vi "Update TDMS Tagged Packet Offsets.vi"(0 "llp tagged packet file path":path, 11 "error in":errorcluster) -> (4 "llp tagged packet file path out":path, 15 "error out":errorcluster)   [LabVIEW 2023, in "GettingStarted_Common_148X_Host.lvlib"]
uses:
  GettingStarted_Common_148X_Host.lvlib
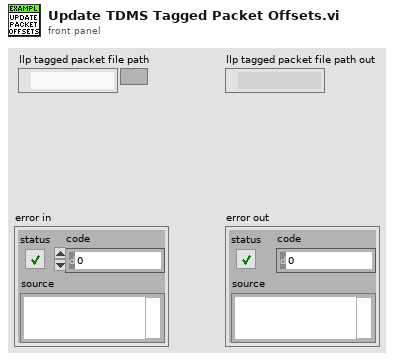
[diagram p1: front panel]
types:
  T1 = enum16{"open", "open or create", "create or replace", "create", "open (read-only)"}
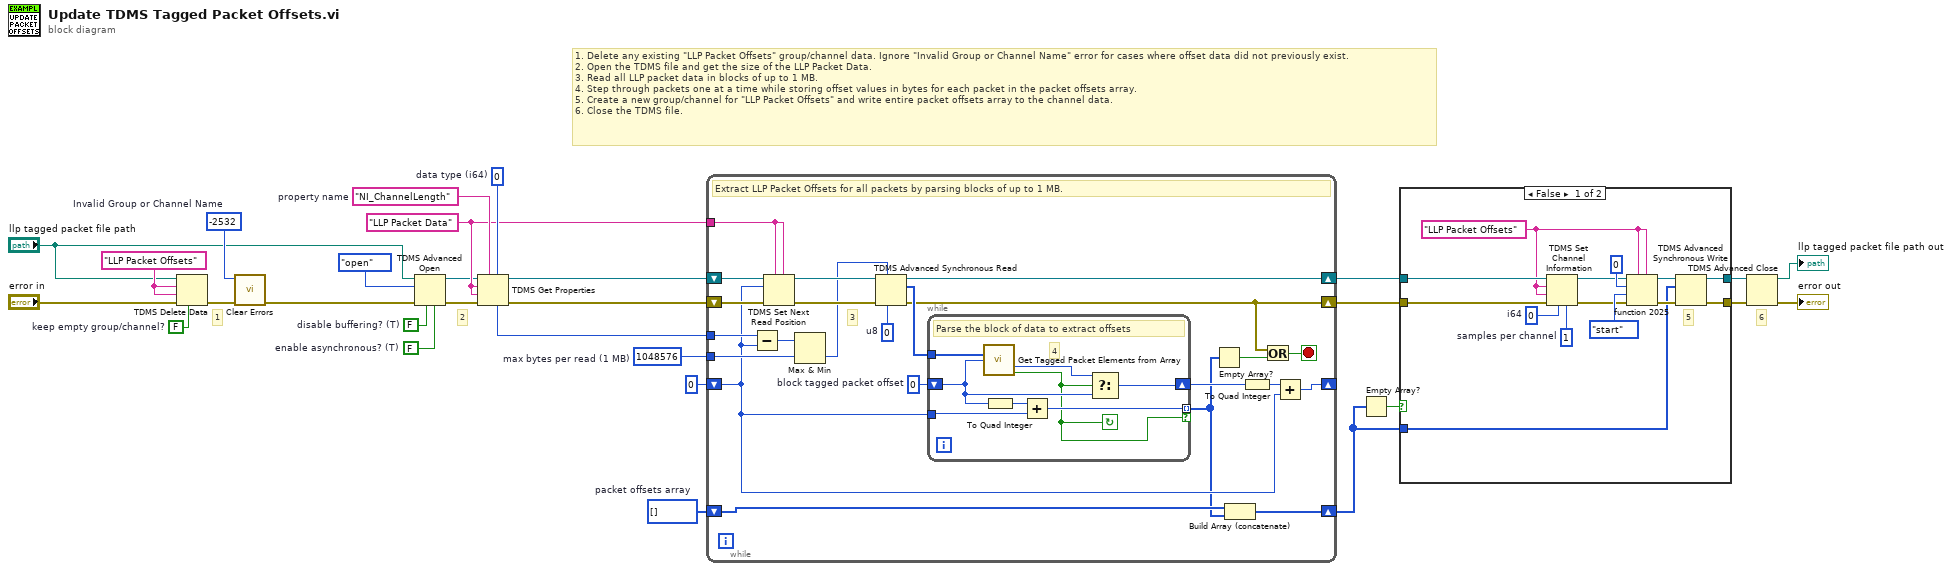
[diagram p0: block diagram]
diagram:
  w2 = -2532  # Invalid Group or Channel Name
  w5 = FALSE  # keep empty group/channel?
  w6 = "LLP Packet Offsets" ("channel and group name")
  w11 = i64[] []  # packet offsets array
  w23 = FALSE  # disable buffering? (T)
  w24 = FALSE  # enable asynchronous? (T)
  w25 = i64 1048576  # max bytes per read (1 MB)
  w28 = i64 0  # data type (i64)
  w29 = "NI_ChannelLength"  # property name
  w27 = "LLP Packet Data" ("channel and group name")
  # "6"
  # "2"
  # "1"
  # "1. Delete any existing \"LLP Packet Offsets\" group/channel data. Ignore \"Invalid Group or Channel Name\" error for cases where offset data did not previously exist.\n2. Open the TDMS file and get the size of the LLP Packet Data.\n3. Read all LLP packet data in blocks of up to 1 MB.\n4. Step through packets one at a time while storing offset values in bytes for each packet in the packet offsets array.\n5. Create a new group/channel for \"LLP Packet Offsets\" and write entire packet offsets array to the channel data.\n6. Close the TDMS file."
  n1 = TDMS Delete Data(6:w5, 8:"error in", 9:w6, 10:w6, 11:"llp tagged packet file path") -> (0:w4:errorcluster)  [unwired: 2 in, 1 out]
  n2 = call <vilib>:"Clear Errors.vi"("error in (no error)"=w4, "specific error code to clear (0: all)"=w2) -> ("error out"=w3:errorcluster)  [unwired: 4 in, 1 out]
  n3 = TDMS Advanced Open(4:w24, 6:w23, 8:w3, 10:T1."open" ("operation (0:open)"), 11:"llp tagged packet file path") -> (0:w13:errorcluster, 3:w12:refnum<k34>)  [unwired: 1 out]
  n4 = TDMS Get Properties(5:w28, 7:w29, 8:w13, 9:w27, 10:w27, 11:w12) -> (0:w19:errorcluster, 3:w18:refnum<k34>, 4:w26:i64)  [unwired: 3 out]
  n5 = while {
    shift-right: [w37] -> w16
    shift-left: w11 -> [w40]
    shift-right: [w36] -> _
    shift-left: i64 0 -> [w34]
    tunnel: w27 -> [w50]
    shift-right: [w31] -> w8
    shift-left: w19 -> [w51]
    shift-right: [w30] -> w9
    shift-left: w18 -> [w52]
    tunnel: w26 -> [w49]
    tunnel: w25 -> [w47]
    stop <- w38 stop-if-true
    w41 = u32 0  # block tagged packet offset
    w43 = u8 0  # u8
    # "3"
    # "Extract LLP Packet Offsets for all packets by parsing blocks of up to 1 MB."
    n6 = Subtract(x=w49, y=w34) -> (x-y=w48:i64)
    n7 = TDMS Set Next Read Position(5:w50, 7:w50, 8:w51, 10:w34, 11:w52) -> (0:w45:errorcluster, 3:w46:refnum<k34>)  [unwired: 1 in]
    n8 = Max & Min(x=w48, y=w47) -> (min(x,y)=w44:i64)  [unwired: 1 out]
    n9 = TDMS Advanced Synchronous Read(6:w43, 7:w44, 8:w45, 11:w46) -> (0:w31:errorcluster, 2:w42:u8[], 3:w30:refnum<k34>)  [unwired: 1 out]
    n10 = while {
      tunnel: w42 -> [w60]
      shift-right: [w56] -> w39
      shift-left: w41 -> [w55]
      tunnel: w34 -> [w54]
      tunnel: [w58] -> w32 mode=indexing if=w53
      stop <- w53 continue-if-true
      # "4"
      # "Parse the block of data to extract offsets"
      n11 = call "Get Tagged Packet Elements from Array.vi"("tagged packet data in"=w60, "tagged packet offset"=w55) -> ("total tagged packet size (bytes)"=w57:u32, "valid packet data?"=w53:bool)  [unwired: 9 in, 3 out]
      n12 = To Quad Integer(1:w55) -> (0:w59:i64)
      n13 = Add(x=w59, y=w54) -> (x+y=w58:i64)
      n14 = Select(t=w57, s=w53, f=w55) -> (s? t:f=w56:u32)
    }
    n15 = Empty Array?(array=w32) -> (empty?=w33:bool)
    n16 = Build Array (concatenate)(w40, w32) -> (w37:i64[])
    n17 = To Quad Integer(1:w39) -> (0:w35:i64)
    n18 = Or(x=w31, y=w33) -> (x .or. y?=w38:bool)
    n19 = Add(x=w35, y=w34) -> (x+y=w36:i64)
  }
  n20 = Empty Array?(array=w16) -> (empty?=w17:bool)
  n21 = case shown="False" w17 {
    tunnel: w9 -> [w65 w76]
    tunnel: w8 -> [w66 w75]
    tunnel: [w73 w76] -> w15
    tunnel: [w74 w75] -> w14
    tunnel: w16 -> [w64 _]
    frame False {
      w61 = "LLP Packet Offsets" ("channel and group name")
      w62 = u32 1  # samples per channel
      w63 = i64 0  # i64
      # "5"
      n22 = TDMS Set Channel Information(4:w62, 6:w63, 8:w66, 9:w61, 10:w61, 11:w65) -> (0:w67:errorcluster, 3:w68:refnum<k34>)  [unwired: 1 in]
      n23 = fn#2025(5:w61, 7:w61, 8:w67, 9:enum16{"start", "end"}."start" ("from (0:start)"), 10:i64 0 ("offset (0)"), 11:w68) -> (0:w70:errorcluster, 3:w69:refnum<k34>)
      n24 = TDMS Advanced Synchronous Write(8:w70, 10:w64, 11:w69) -> (0:w74:errorcluster, 3:w73:refnum<k34>)
    }
    frame True {
    }
  }
  n25 = TDMS Advanced Close(8:w14, 11:w15) -> (0:→"error out":errorcluster, 3:→"llp tagged packet file path out":path)  [unwired: 2 in]
